vi "Read Multiple Digital Inputs.vi"(0 "Lines":tag, 5 "Expected Array":bool[](array[boolean]), 11 "Error In":errorcluster) -> (4 "Pass/Fail?":bool, 6 "Report Text":string, 8 "Actual Array":bool[](array[boolean]), 15 "Error Out":errorcluster)   [LabVIEW 2016]
doc: "This VI reads multiple digital input lines and compares these values to an array of expected values, with pass/fail and report text outputs."
uses:
  <vilib>/DAQmx/read.llb/DAQmx Read (Digital 1D Bool NChan 1Samp 1Line).vi
  <vilib>/DAQmx/create/channels.llb/DAQmx Create Channel (DI-Digital Input).vi
  <vilib>/DAQmx/miscellaneous.llb/DAQmx Fill In Error Info.vi
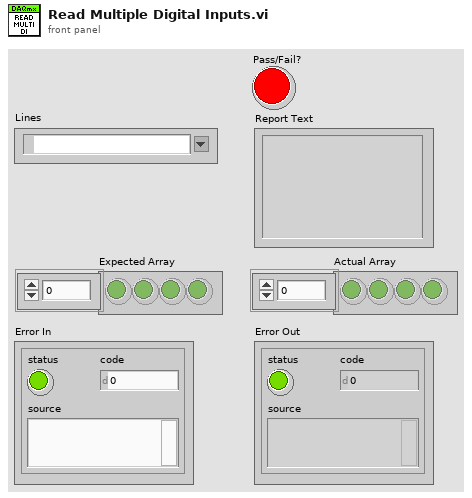
[diagram p1: front panel]
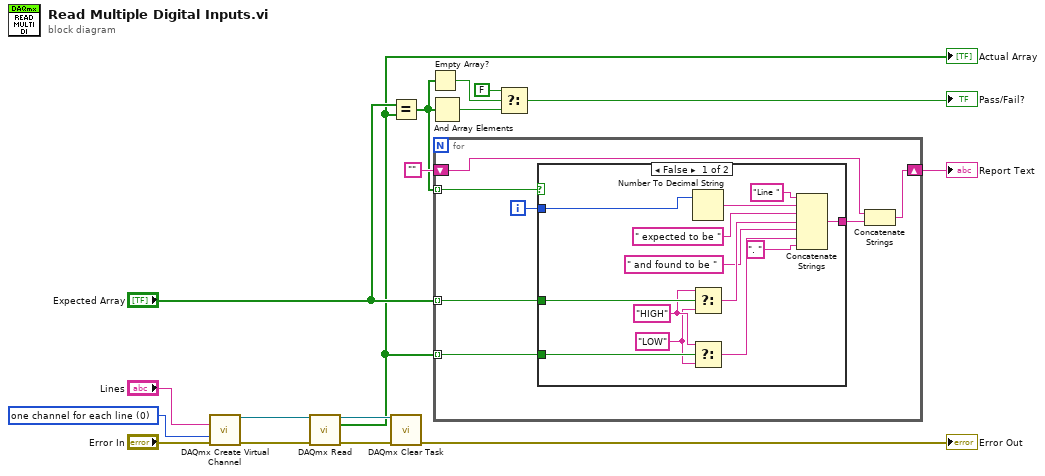
[diagram p0: block diagram]
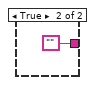
[diagram p2: hidden frame]
diagram:
  w17 = 0 items=["one channel for each line", "one channel for all lines"] ("line grouping")
  n1 = call-poly <vilib>:"DAQmx Create Virtual Channel.vi"("lines"="Lines", "line grouping"=w17, "error in"="Error In") -> ("task out"=w13:refnum<k21>, "error out"=w16:errorcluster)  [unwired: 11 in]
  n2 = call-poly <vilib>:"DAQmx Read.vi"("task/channels in"=w13, "error in"=w16) -> ("task out"=w14:refnum<k21>, "data"=w8:bool[], "error out"=w15:errorcluster)  [unwired: 11 in]
  "Actual Array" <- w8
  n3 = Equal?(x="Expected Array", y=w8) -> (x = y?=w5:bool[])
  n4 = call <vilib>:"DAQmx Clear Task.vi"("task in"=w14, "error in"=w15) -> ("error out"=→"Error Out":errorcluster)  [unwired: 13 in]
  n5 = Empty Array?(array=w5) -> (empty?=w4:bool)
  n6 = And Array Elements(Boolean array=w5) -> (logical AND=w2:bool)
  n7 = for {
    tunnel: w8 -> [w24] mode=indexing
    tunnel: "Expected Array" -> [w23] mode=indexing
    tunnel: w5 -> [w22] mode=indexing
    shift-right: [w20] -> w7
    shift-left: "" -> [w19]
    i -> [w18]
    n8 = case shown="False" w22 {
      tunnel: w23 -> [w37 _]
      tunnel: w24 -> [w36 _]
      tunnel: [w31 ""] -> w21
      tunnel: w18 -> [w27 _]
      frame False {
        w29 = "LOW" ("Report Text")
        w30 = "HIGH" ("Report Text")
        n9 = Number To Decimal String(number=w27) -> (decimal integer string=w26:string)  [unwired: 1 in]
        n10 = Select(t=w30, s=w37, f=w29) -> (s? t:f=w34:string)
        n11 = Select(t=w30, s=w36, f=w29) -> (s? t:f=w32:string)
        n12 = Concatenate Strings("Line " ("string"), w26, " expected to be " ("string"), w34, " and found to be " ("string"), w32, ". ") -> (w31:string)
      }
      frame True {
      }
    }
    n13 = Concatenate Strings(w19, w21) -> (w20:string)
  }
  "Report Text" <- w7
  n14 = Select(t=FALSE, s=w4, f=w2) -> (s? t:f=→"Pass/Fail?":bool)
